vi "LJUD_TCVoltsToTemp.vi"(7 "TCType":i32=6004, 8 "error in":errorcluster, 9 "CJTempK":dbl format="%.2f", 10 "TCVolts":dbl format="%.4f") -> (0 "error out":errorcluster, 1 "TCTempF":dbl format="%.2f", 2 "TCTempC":dbl format="%.2f", 3 "TCTempK":dbl format="%.2f")   [LabVIEW 2021]
uses:
  labjackud.dll
panel:
  # "Requires UD driver V2.60+."
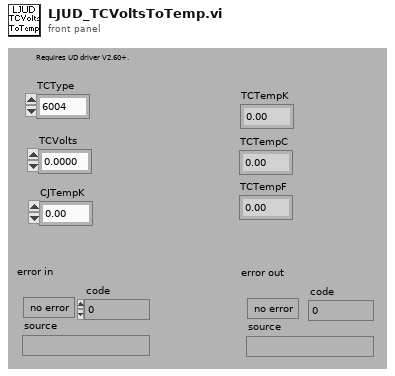
[diagram p1: front panel]
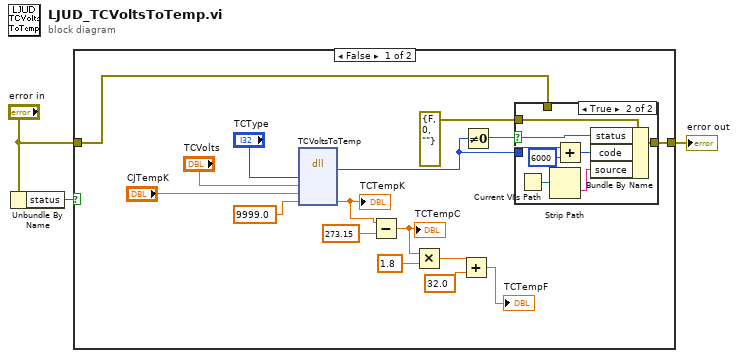
[diagram p0: block diagram]
diagram:
  n1 = Unbundle By Name("error in") -> ("status"=w2:bool)
  n2 = case shown="False" w2 {
    tunnel: [w16 w29] -> w3
    tunnel: "error in" -> [w15 w29]
    frame False {
      n3 = dll-call lib="labjackud.dll" fn="TCVoltsToTemp"("TCType"="TCType", "TCVolts"="TCVolts", "CJTempK"="CJTempK", "TCTempK"=9999.0) -> (w17:i32, "TCTempK"=w7:dbl)  [unwired: 6 in, 2 out]
      "TCTempK" <- w7
      n4 = Subtract(x=w7, y=273.15) -> (x-y=w6:dbl)
      "TCTempC" <- w6
      n5 = Multiply(x=w6, y=1.8) -> (x*y=w5:dbl)
      n6 = Add(x=w5, y=32.0) -> (x+y=→"TCTempF":dbl)
      n7 = Not Equal To 0?(x=w17) -> (x != 0?=w18:bool)
      n8 = case shown="True" w18 {
        selector: w18 -> [_ w27]
        tunnel: [w20 w28] -> w16
        tunnel: errorcluster {"status"=FALSE, "code"=0, "source"=""} ("error IO") -> [_ w26]
        tunnel: w17 -> [_ w22]
        tunnel: w15 -> [w20 _]
        frame False {
        }
        frame True {
          n9 = Current VI's Path() -> (path=w24:path)
          n10 = Strip Path(path=w24) -> (name=w25:string)  [unwired: 1 out]
          n11 = Add(x=w22, y=6000) -> (x+y=w23:i32)
          n12 = Bundle By Name(cluster=w26, "status"=w27, "code"=w23, "source"=w25) -> (w28:errorcluster)
        }
      }
    }
    frame True {
    }
  }
  "error out" <- w3
